vi "fileUpTempWithSN&Date_copy.vi"(0 "DateCode默认类型":string, 2 "DateCode默认类型：":enum16{"0X20", "0X30", "0X00"}(ring), 4 "校验信息":T1(array[cluster]), 5 "input_str_customer":string, 6 "input_str_SN":string, 7 "input_str_Date":string, 8 "input_array_temp_int":u8[][](array[numeric]) format="%.0x") -> (1 "Output String":string[](array[string]), 3 "show_array_temp_int":u8[][](array[numeric])=[[3, 4, 33, 0, 0, 0, 0, 65, 4, 128, 213, 0, 103, 0, 0, 0, 0, 0, 0, 0, 0, 0, 0, 0, 0, 0, 0, 0, 0, 0, 0, 0, 0, 0, 0, 0, 0, 0, 0, 0, 0, 0, 0, 0, 0, 0, 0, 0, 0, 0, 0, 0, 0, 0, 0, 0, 0, 0, 0, 0, 1, 0, 0, 42, 0, 0, 0, 0, 0, 0, 0, 0, 0, 0, 0, 0, 0, 0, 0, 0, 0, 0, 0, 0, 49, 52, 49, 49, 50, 53, 0, 0, 0, 0, 0, 46, 0, 0, 0, 0, 0, 0, 0, 0, 0, 0, 0, 0, 0, 0, 0, 0, 0, 0, 0, 0, 0, 0, 0, 0, 0, 0, 0, 0, 0, 0, 0, 0, 0, 0, 0, 0, 0, 0, 0, 0, 0, 0, 0, 0, 0, 0, 0, 0, 0, 0, 0, 0, 0, 0, 0, 0, 0, 0, 0, 0, 0, 0, 0, 0, 0, 0, 0, 0, 0, 0, 0, 0, 0, 0, 0, 0, 0, 0, 0, 0, 0, 0, 0, 0, 0, 0, 0, 0, 0, 0, 0, 0, 0, 0, 0, 0, 0, 0, 0, 0, 0, 0, 0, 0, 0, 0, 0, 0, 0, 0, 0, 0, 0, 0, 0, 0, 0, 0, 0, 0, 0, 0, 0, 0, 0, 0, 0, 0, 0, 0, 0, 0, 0, 0, 0, 0, 0, 0, 0, 0, 0, 0, 0, 0, 0, 0, 0, 0, 0, 0, 0, 0, 0, 0, 0, 0, 0, 0, 0, 0]] format="%.0x")   [LabVIEW 2011]
panel:
  # "file up template with SN and Date"
  # "If this Switch is True,then Datecode 8 bit default is 0X30,If the Switch is fail ,the datecode 8 bit are 0X20"
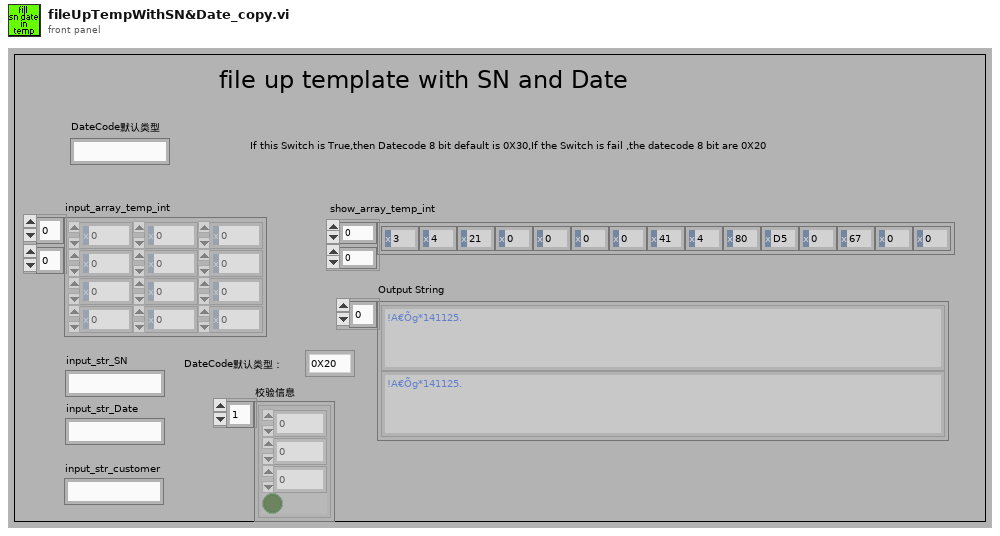
[diagram p1: front panel]
types:
  T1 = cluster{"start":i32, "length":i32, "p":i32, "H/L":bool}[]
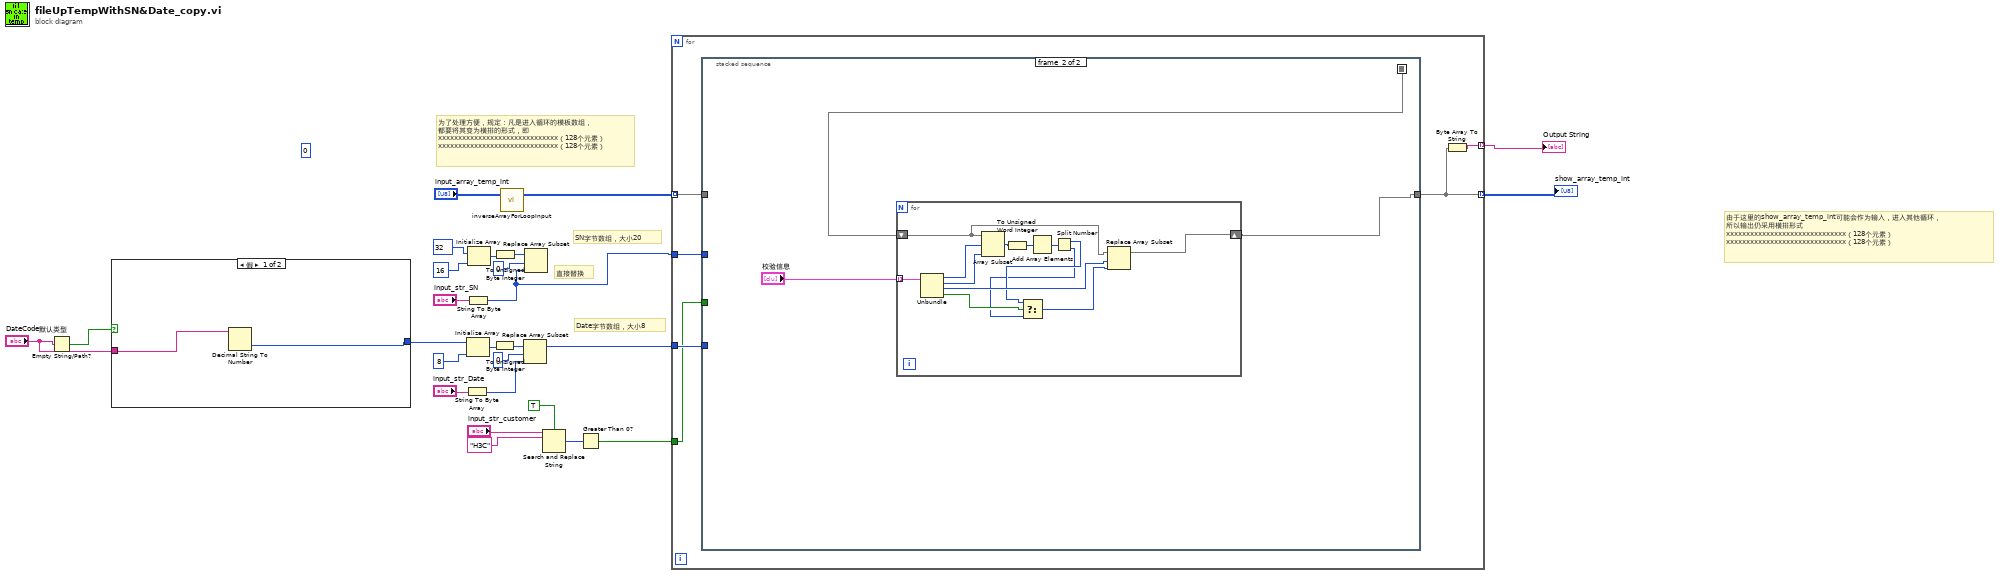
[diagram p0: block diagram]
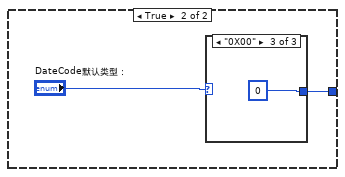
[diagram p2: hidden frame]
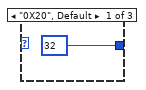
[diagram p3: hidden frame]
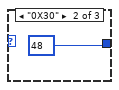
[diagram p4: hidden frame]
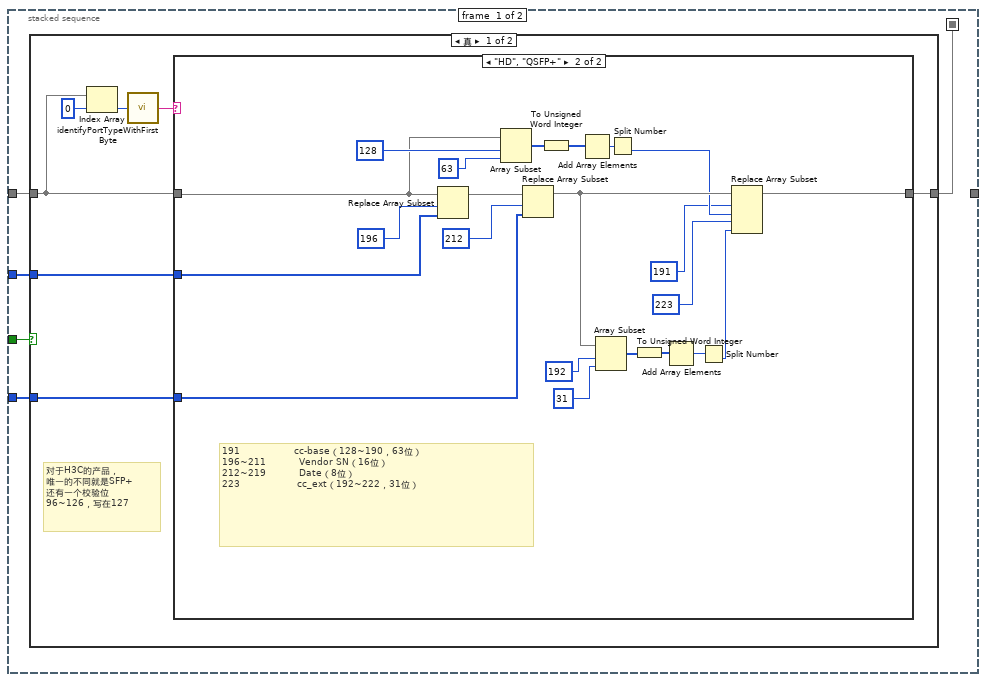
[diagram p5: hidden frame]
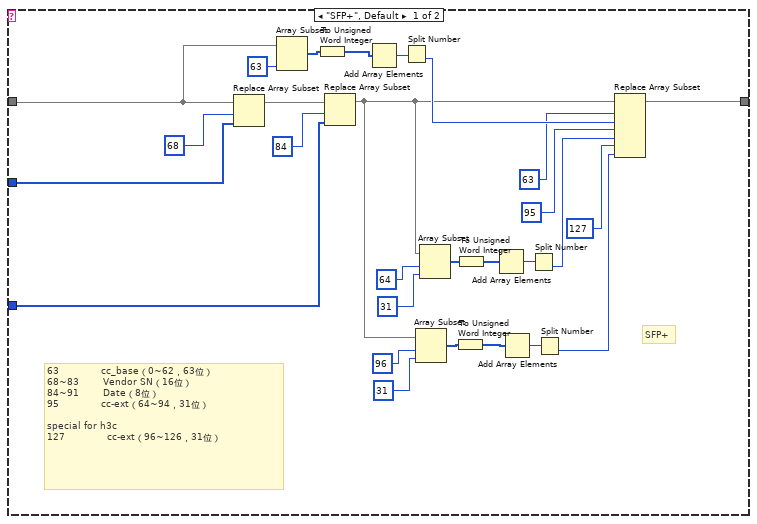
[diagram p6: hidden frame]
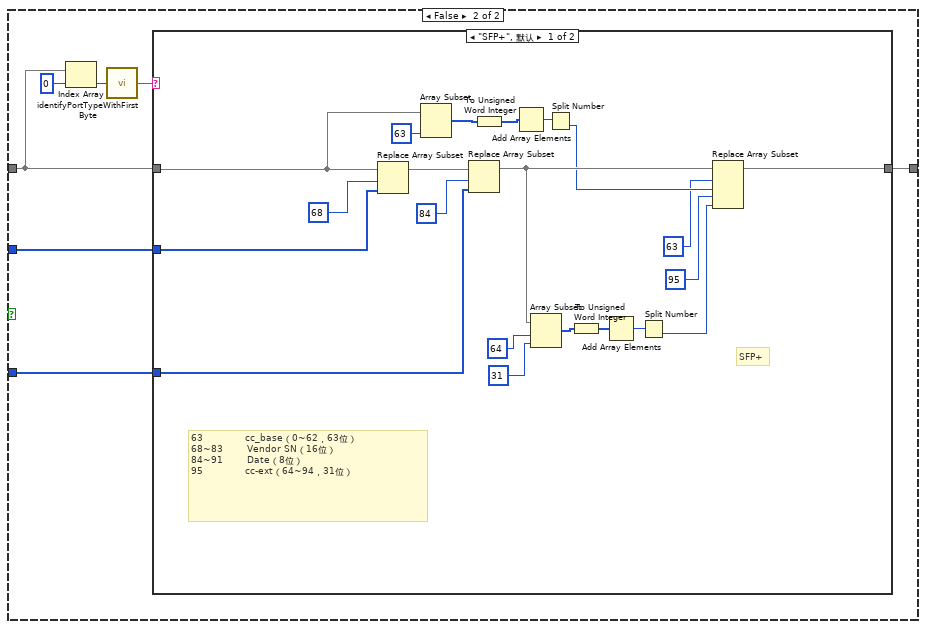
[diagram p7: hidden frame]
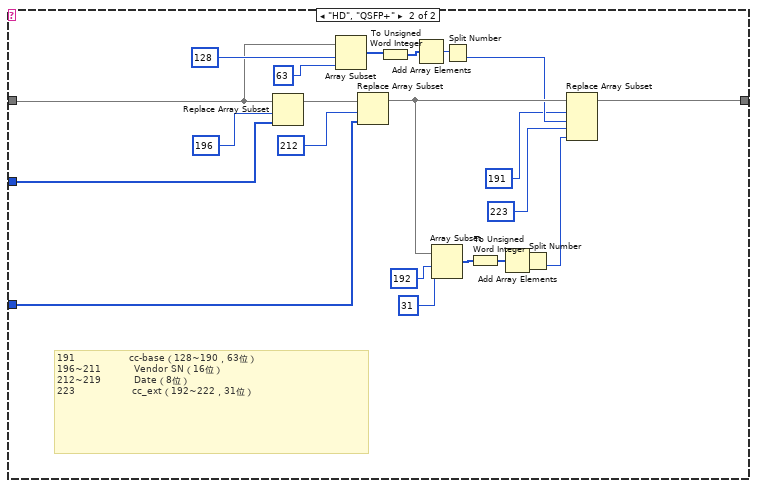
[diagram p8: hidden frame]
diagram:
  (unwired) 0
  # "直接替换"
  # "由于这里的show_array_temp_int可能会作为输入，进入其他循环，\n所以输出仍采用横排形式\nxxxxxxxxxxxxxxxxxxxxxxxxxxxxxx（128个元素）\nxxxxxxxxxxxxxxxxxxxxxxxxxxxxxx（128个元素）"
  # "Date字节数组，大小8"
  # "SN字节数组，大小20"
  # "为了处理方便，规定：凡是进入循环的模板数组，\n都要将其变为横排的形式，即\nxxxxxxxxxxxxxxxxxxxxxxxxxxxxxx（128个元素）\nxxxxxxxxxxxxxxxxxxxxxxxxxxxxxx（128个元素）"
  n1 = Empty String/Path?(string/path="DateCode默认类型") -> (empty?=w3:bool)
  n2 = case shown="假" w3 {
    tunnel: [w27 w30] -> w4
    tunnel: "DateCode默认类型" -> [w28 _]
    frame False {
      n3 = Decimal String To Number(string=w28) -> (number=w27:i32)  [unwired: 2 in, 1 out]
    }
    frame True {
      n4 = case shown="\"0X00\"" "DateCode默认类型：" {
        tunnel: [32 48 0] -> w30
        frame "0X20", Default {
        }
        frame "0X30" {
        }
        frame "0X00" {
        }
      }
    }
  }
  n5 = String To Byte Array(string="input_str_Date") -> (unsigned byte array=w18:u8[])
  n6 = String To Byte Array(string="input_str_SN") -> (unsigned byte array=w1:u8[])
  n7 = Initialize Array(w4, 8 ("维数大小")) -> (w16:i32[])
  n8 = Initialize Array(32, 16 ("维数大小")) -> (w22:i32[])
  n9 = To Unsigned Byte Integer(number=w16) -> (unsigned 8bit integer=w17:u8[])
  n10 = To Unsigned Byte Integer(number=w22) -> (unsigned 8bit integer=w21:u8[])
  n11 = call "inverseArrayForLoopInput.vi"("input_array_temp_int"="input_array_temp_int") -> ("show_array_temp_int"=w25:u8[][])  [unwired: 1 in, 1 out]
  n12 = Replace Array Subset(array=w17, new element=w18, index=0 ("索引")) -> (w13:u8[])
  n13 = Replace Array Subset(array=w21, new element=w1, index=0 ("索引")) -> ()  [unwired: 1 out]
  n14 = Search and Replace String(case sensitive?=TRUE ("忽略大小写？(F)"), input string="input_str_customer", search string="H3C" ("搜索字符串")) -> (number of replacements=w7:i32)  [unwired: 5 in, 3 out]
  n15 = Greater Than 0?(x=w7) -> (x > 0?=w6:bool)
  n16 = for {
    tunnel: w25 -> [w39] mode=indexing
    tunnel: w1 -> [w38]
    tunnel: w13 -> [w37]
    tunnel: [w36] -> w12 mode=indexing
    tunnel: [w35] -> w11 mode=indexing
    tunnel: w6 -> [w34]
    n17 = stacked-sequence {
      seq-local: [w40 _] -> [_ w153]
      tunnel: w39 -> [w44 _]
      tunnel: w38 -> [w43 _]
      tunnel: w37 -> [w42 _]
      tunnel: [_ w152] -> w36
      tunnel: w34 -> [w41 _]
      frame #0 {
        n18 = case shown="真" w41 {
          tunnel: w44 -> [w48 w105]
          tunnel: w43 -> [w47 w104]
          tunnel: w42 -> [w46 w103]
          tunnel: [w45 w102] -> w40
          frame True {
            # "对于H3C的产品，\n唯一的不同就是SFP+\n还有一个校验位\n96~126，写在127"
            n19 = Index Array(array=w48, index=0 ("索引")) -> (element=w50:u8)
            n20 = call "identifyPortTypeWithFirstByte.vi"("input_int"=w50) -> ("show_str_portType"=w49:string)
            n21 = case shown="\"HD\", \"QSFP+\"" w49 {
              tunnel: w48 -> [w67 w87]
              tunnel: w47 -> [w66 w86]
              tunnel: w46 -> [w65 w85]
              tunnel: [w64 w84] -> w45
              frame "SFP+", Default {
                # "63              cc_base（0~62，63位）\n68~83        Vendor SN（16位）\n84~91        Date（8位）\n95              cc-ext（64~94，31位）\n\nspecial for h3c\n127              cc-ext（96~126，31位）"
                # "SFP+"
                n22 = Replace Array Subset(array=w67, new element=w66, index=68 ("索引")) -> (w74:u8[])
                n23 = Array Subset(array=w67, length=63 ("长度")) -> (w57:u8[])  [unwired: 1 in]
                n24 = To Unsigned Word Integer(number=w57) -> (unsigned 16bit integer=w56:u16[])
                n25 = Replace Array Subset(array=w74, new element=w65, index=84 ("索引")) -> (w60:u8[])
                n26 = Add Array Elements(numeric array=w56) -> (sum=w73:u16)
                n27 = Split Number(x=w73) -> (lo(x)=w75:u8)  [unwired: 1 out]
                n28 = Array Subset(array=w60, index=96 ("索引"), length=31 ("长度")) -> (w53:u8[])
                n29 = Array Subset(array=w60, index=64 ("索引"), length=31 ("长度")) -> (w55:u8[])
                n30 = To Unsigned Word Integer(number=w53) -> (unsigned 16bit integer=w52:u16[])
                n31 = To Unsigned Word Integer(number=w55) -> (unsigned 16bit integer=w54:u16[])
                n32 = Add Array Elements(numeric array=w54) -> (sum=w77:u16)
                n33 = Add Array Elements(numeric array=w52) -> (sum=w62:u16)
                n34 = Split Number(x=w77) -> (lo(x)=w79:u8)  [unwired: 1 out]
                n35 = Split Number(x=w62) -> (lo(x)=w59:u8)  [unwired: 1 out]
                n36 = Replace Array Subset(array=w60, new element #1=w75, index #1=63 ("索引"), new element #2=w79, index #2=95 ("索引"), new element #3=w59, index #3=127 ("索引")) -> (w64:u8[])
              }
              frame "HD", "QSFP+" {
                # "191                  cc-base（128~190，63位）\n196~211           Vendor SN（16位）\n212~219           Date（8位）\n223                   cc_ext（192~222，31位）"
                n37 = Replace Array Subset(array=w87, new element=w86, index=196 ("索引")) -> (w94:u8[])
                n38 = Array Subset(array=w87, index=128 ("长度"), length=63 ("长度")) -> (w83:u8[])
                n39 = Replace Array Subset(array=w94, new element=w85, index=212 ("索引")) -> (w99:u8[])
                n40 = To Unsigned Word Integer(number=w83) -> (unsigned 16bit integer=w82:u16[])
                n41 = Add Array Elements(numeric array=w82) -> (sum=w93:u16)
                n42 = Array Subset(array=w99, index=192 ("索引"), length=31 ("长度")) -> (w81:u8[])
                n43 = Split Number(x=w93) -> (lo(x)=w95:u8)  [unwired: 1 out]
                n44 = To Unsigned Word Integer(number=w81) -> (unsigned 16bit integer=w80:u16[])
                n45 = Add Array Elements(numeric array=w80) -> (sum=w97:u16)
                n46 = Split Number(x=w97) -> (lo(x)=w100:u8)  [unwired: 1 out]
                n47 = Replace Array Subset(array=w99, new element #1=w95, index #1=191 ("索引"), new element #2=w100, index #2=223 ("索引")) -> (w84:u8[])
              }
            }
          }
          frame False {
            n48 = Index Array(array=w105, index=0 ("索引")) -> (element=w107:u8)
            n49 = call "identifyPortTypeWithFirstByte.vi"("input_int"=w107) -> ("show_str_portType"=w106:string)
            n50 = case shown="\"SFP+\", 默认" w106 {
              tunnel: w105 -> [w116 w137]
              tunnel: w104 -> [w115 w136]
              tunnel: w103 -> [w114 w135]
              tunnel: [w113 w134] -> w102
              frame "SFP+", Default {
                # "63              cc_base（0~62，63位）\n68~83        Vendor SN（16位）\n84~91        Date（8位）\n95              cc-ext（64~94，31位）"
                # "SFP+"
                n51 = Replace Array Subset(array=w116, new element=w115, index=68 ("索引")) -> (w123:u8[])
                n52 = Array Subset(array=w116, length=63 ("长度")) -> (w112:u8[])  [unwired: 1 in]
                n53 = Replace Array Subset(array=w123, new element=w114, index=84 ("索引")) -> (w128:u8[])
                n54 = To Unsigned Word Integer(number=w112) -> (unsigned 16bit integer=w111:u16[])
                n55 = Add Array Elements(numeric array=w111) -> (sum=w122:u16)
                n56 = Array Subset(array=w128, index=64 ("索引"), length=31 ("长度")) -> (w110:u8[])
                n57 = Split Number(x=w122) -> (lo(x)=w124:u8)  [unwired: 1 out]
                n58 = To Unsigned Word Integer(number=w110) -> (unsigned 16bit integer=w109:u16[])
                n59 = Add Array Elements(numeric array=w109) -> (sum=w126:u16)
                n60 = Split Number(x=w126) -> (lo(x)=w129:u8)  [unwired: 1 out]
                n61 = Replace Array Subset(array=w128, new element #1=w124, index #1=63 ("索引"), new element #2=w129, index #2=95 ("索引")) -> (w113:u8[])
              }
              frame "HD", "QSFP+" {
                # "191                  cc-base（128~190，63位）\n196~211           Vendor SN（16位）\n212~219           Date（8位）\n223                   cc_ext（192~222，31位）"
                n62 = Replace Array Subset(array=w137, new element=w136, index=196 ("索引")) -> (w144:u8[])
                n63 = Array Subset(array=w137, index=128 ("长度"), length=63 ("长度")) -> (w133:u8[])
                n64 = Replace Array Subset(array=w144, new element=w135, index=212 ("索引")) -> (w149:u8[])
                n65 = To Unsigned Word Integer(number=w133) -> (unsigned 16bit integer=w132:u16[])
                n66 = Add Array Elements(numeric array=w132) -> (sum=w143:u16)
                n67 = Array Subset(array=w149, index=192 ("索引"), length=31 ("长度")) -> (w131:u8[])
                n68 = Split Number(x=w143) -> (lo(x)=w145:u8)  [unwired: 1 out]
                n69 = To Unsigned Word Integer(number=w131) -> (unsigned 16bit integer=w130:u16[])
                n70 = Add Array Elements(numeric array=w130) -> (sum=w147:u16)
                n71 = Split Number(x=w147) -> (lo(x)=w150:u8)  [unwired: 1 out]
                n72 = Replace Array Subset(array=w149, new element #1=w145, index #1=191 ("索引"), new element #2=w150, index #2=223 ("索引")) -> (w134:u8[])
              }
            }
          }
        }
      }
      frame #1 {
        n73 = for {
          tunnel: "校验信息" -> [w167] mode=indexing
          shift-right: [w157] -> w152
          shift-left: w153 -> [w163]
          n74 = Unbundle(w167) -> ("start"=w165:i32, "length"=w164:i32, "p"=w162:i32, "H/L"=w161:bool)
          n75 = Array Subset(array=w163, index=w165, length=w164) -> (w156:u8[])
          n76 = To Unsigned Word Integer(number=w156) -> (unsigned 16bit integer=w155:u16[])
          n77 = Add Array Elements(numeric array=w155) -> (sum=w166:u16)
          n78 = Split Number(x=w166) -> (hi(x)=w160:u8, lo(x)=w159:u8)
          n79 = Select(t=w160, s=w161, f=w159) -> (s? t:f=w158:u8)
          n80 = Replace Array Subset(array=w163, new element=w158, index=w162) -> (w157:u8[])
        }
      }
    }
    n81 = Byte Array To String(unsigned byte array=w36) -> (string=w35:string)
  }
  "show_array_temp_int" <- w12
  "Output String" <- w11
